vi "PH_SRDG645.Read DB.vi"(0 "i ref in":refnum<vi>, 5 "error in":errorcluster) -> (14 "i ref out":refnum<vi>, 16 "Default Name":string, 19 "error out":errorcluster)   [LabVIEW 2014, in "PH_SRDG645.lvlib"]
doc: "This VI reads out relevant data base information and writes it to own attributes and the GUI."
uses:
  PH_SRDG645.lvlib
  PH_Basics/PH_Common/PH_Common.lvlib
  CS_Core/CSSystem/CSSystemLib/CSSystemLib.lvlib
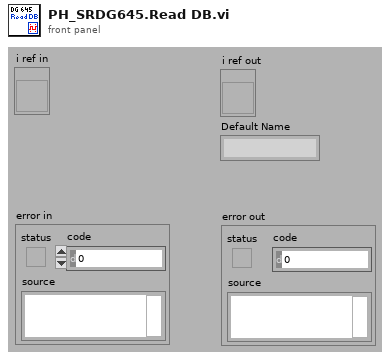
[diagram p1: front panel]
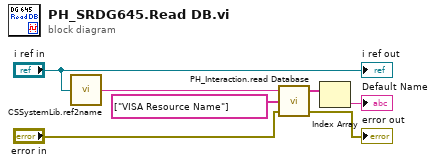
[diagram p0: block diagram]
diagram:
  n1 = call "CSSystemLib.ref2name.vi"("obj refnum"="i ref in") -> ("name"=w6:string)
  n2 = call "PH_Interaction.read Database.vi"("error in (no error)"="error in", "Strings to search for"=string[] ["VISA Resource Name"], "DB Entry to read"=w6) -> ("error out"=→"error out":errorcluster, "Values"=w7:string[])  [unwired: 1 in]
  n3 = Index Array(array=w7) -> (element=→"Default Name":string)  [unwired: 1 in]
  "i ref out" <- "i ref in"
